vi "Advance Query Adjust In built table.vi"(8 "error in (no error)":errorcluster, 10 "Database in":refnum<class "Database.lvclass">, 11 "PluginWithDatabase":refnum<class "PluginWithDatabase.lvclass">) -> (0 "error out":errorcluster, 3 "PluginWithDatabase out":refnum<class "PluginWithDatabase.lvclass">)   [LabVIEW 2015, in "ActorManagement.lvlib" / "PluginWithDatabase.lvclass"]
uses:
  PluginWithDatabase.lvclass
  DatabaseManagement/Database.lvclass
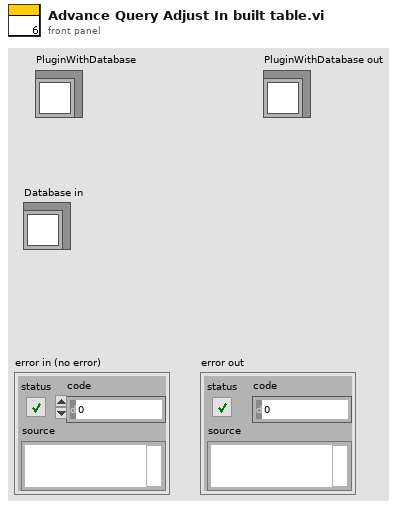
[diagram p1: front panel]
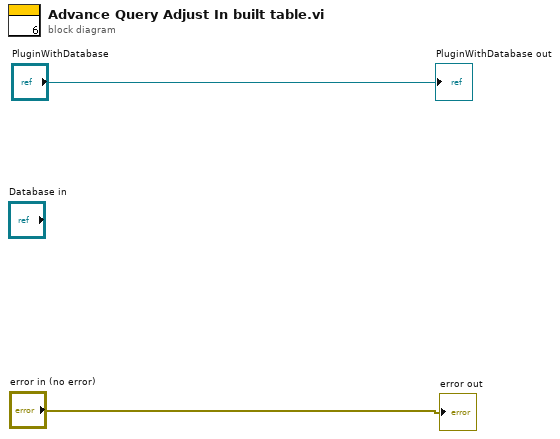
[diagram p0: block diagram]
diagram:
  "error out" <- "error in (no error)"
  "PluginWithDatabase out" <- "PluginWithDatabase"
